vi "Read Attribute Meta Data.vi"(7 "Linked List ID":string, 8 "error in (no error)":errorcluster, 9 "Attribute Type":variant, 10 "Attribute Name":string, 11 "Linked List Ref":refnum<data-value>) -> (0 "error out":errorcluster, 1 "Found?":bool, 3 "Linked List Ref out":refnum<data-value>, 6 "Meta Data":string)   [LabVIEW 2020, in "Linked Lists.lvlib" / "Linked List Ref.lvclass"]
uses:
  <vilib>/gpm_packages/@cs/linked-list/Source/Linked List/Linked List Ref/Linked List Ref.lvclass
  <vilib>/gpm_packages/@cs/linked-list/Source/Linked List/ILinkedList/ILinked List.lvclass
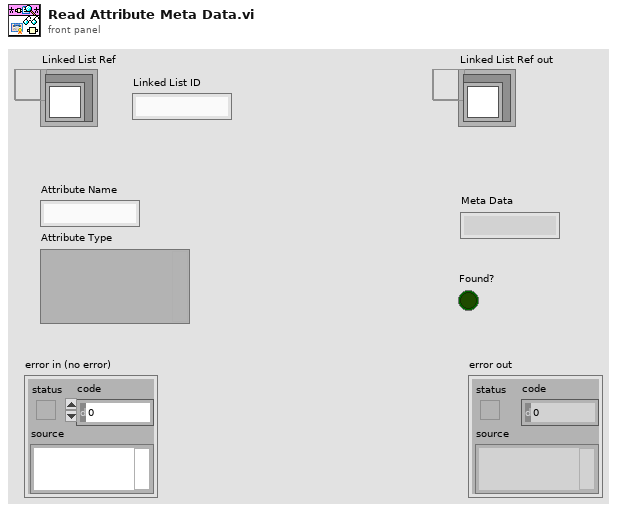
[diagram p1: front panel]
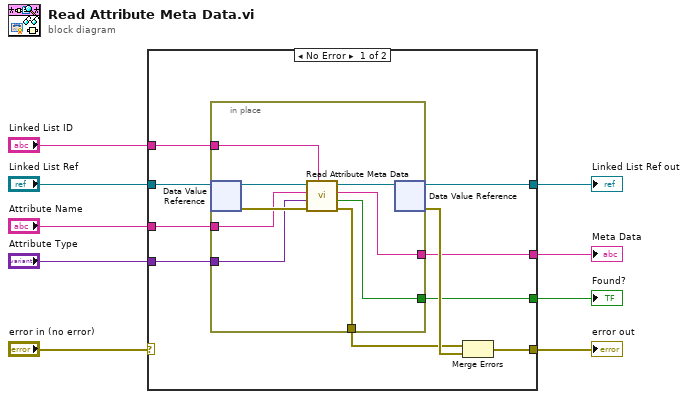
[diagram p0: block diagram]
diagram:
  n1 = case shown="No Error" "error in (no error)" {
    selector: "error in (no error)" -> [_ w30]
    tunnel: "Linked List Ref" -> [w19 w29]
    tunnel: "Linked List ID" -> [w18 _]
    tunnel: [w16 w30] -> w6
    tunnel: [w17 w29] -> w5
    tunnel: "Attribute Name" -> [w13 _]
    tunnel: "Attribute Type" -> [w12 _]
    tunnel: [w11 _] -> w2
    tunnel: [w10 _] -> w1
    frame No Error {
      n2 = in-place {
        in-place-border: w18 -> [w24]
        in-place-border: [w25] -> w14
        in-place-border: w13 -> [w23]
        in-place-border: w12 -> [w22]
        in-place-border: [w21] -> w11
        in-place-border: [w20] -> w10
        n3 = in-place-dvr #1(w19) -> (w28:refnum<class "ILinked List.lvclass">, w26:errorcluster)
        n4 = call-dynamic "Read Attribute Meta Data.vi"("Linked List ID"=w24, "error in (no error)"=w26, "Attribute Type"=w22, "Attribute Name"=w23, "ILinked List in"=w28) -> ("error out"=w25:errorcluster, "Found?"=w21:bool, "Meta Data"=w20:string, "ILinked List out"=w27:refnum<class "ILinked List.lvclass">)  [unwired: 3 in]
        n5 = in-place-dvr #1(w27) -> (w17:refnum<data-value>, w15:errorcluster)
      }
      n6 = Merge Errors(w14, w15) -> (w16:errorcluster)
    }
    frame Error {
    }
  }
  "error out" <- w6
  "Linked List Ref out" <- w5
  "Meta Data" <- w1
  "Found?" <- w2
